vi "Clear Task.vi"(8 "error in (no error)":errorcluster, 11 "DAQmx Actor in":refnum<class "DAQmx Actor.lvclass">) -> (0 "error out":errorcluster, 3 "DAQmx Actor out":refnum<class "DAQmx Actor.lvclass">)   [LabVIEW 2024, in "DAQmx Actor.lvlib" / "DAQmx Actor.lvclass"]
uses:
  DAQmx Actor.lvclass
  DAQmx Actor.lvclass/DAQmx Actor.ctl
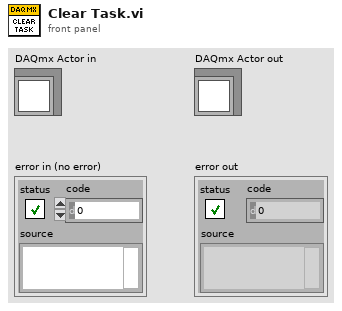
[diagram p1: front panel]
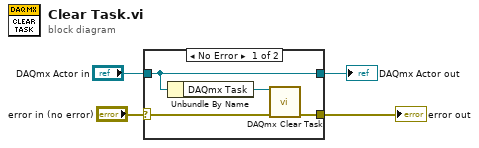
[diagram p0: block diagram]
diagram:
  n1 = case shown="No Error" "error in (no error)" {
    selector: "error in (no error)" -> [w6 w10]
    tunnel: [w5 w10] -> w3
    tunnel: [w8 w9] -> w1
    tunnel: "DAQmx Actor in" -> [w8 w9]
    frame No Error {
      n2 = Unbundle By Name(w8) -> ("DAQmx Task"=w7:refnum<k21>)
      n3 = call <vilib>:"DAQmx Clear Task.vi"("task in"=w7, "error in"=w6) -> ("error out"=w5:errorcluster)  [unwired: 13 in]
    }
    frame Error {
    }
  }
  "error out" <- w3
  "DAQmx Actor out" <- w1
